vi "_FPGA Wait.vi"(4 "error in":errorcluster, 5 "Timeout (2000ms)":u32=2000, 6 "Indicator":T1=enum."Ready") -> (0 "error out":errorcluster)   [LabVIEW 2012]
uses:
  Type/_FPGA Indicator.ctl
  Type/_RW Status.ctl
  Type/_LED States.ctl
  _RT Global.vi
  <vilib>/Utility/error.llb/Error Cluster From Error Code.vi
  <vilib>/rvi/errors/niLvFpgaAdjustHostInterfaceError.vi
  <vilib>/rvi/interface/nirviReadWriteControl/nirviReadWriteControl.xnode
  FPGA Bitfiles/FPGA9606.lvbitx
  NiFpgaLv.dll
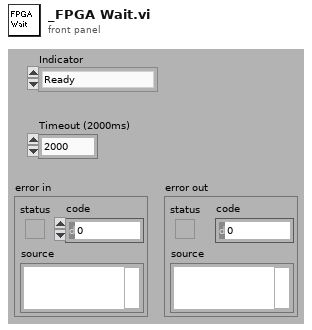
[diagram p1: front panel]
types:
  T1 = typedef "_FPGA Indicator.ctl" = enum16{"Done", "Ready", "Count Available", "SendSerial", "LED State"}
  T2 = typedef "_RW Status.ctl" = enum8{"Done", "Do Read", "Do Write", "Set Latch1", "Set Latch2", "Set Latch3", "Set Latch4", "RP ON", "EL ON", "Serial Send", "Set LC Out", "Get LC In", "Read VAC", "Table Test", "Get Interlock", "Do Read2", "Do Write2"}
  T3 = typedef "_LED States.ctl" = enum8{"Idle", "Solid B", "Solid R", "Solid P", "Off B", "Off R", "Off P", "Off BRP", "Off RP", "Flash R&P", "Flash P"}
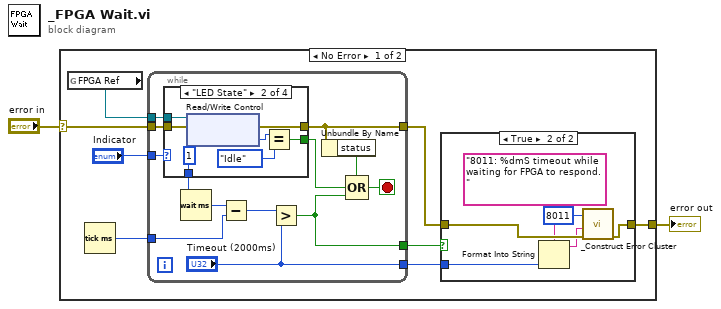
[diagram p0: block diagram]
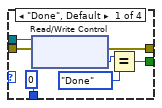
[diagram p3: hidden frame]
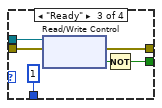
[diagram p4: hidden frame]
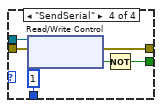
[diagram p5: hidden frame]
diagram:
  n1 = case shown="No Error" "error in" {
    selector: "error in" -> [w5 w56]
    tunnel: [w7 w56] -> w2
    frame No Error {
      n2 = global read "_RT Global.vi" "FPGA Ref"() -> (w3:refnum<k20>)
      n3 = Tick Count (ms)() -> (millisecond timer value=w10:u32)
      n4 = while {
        tunnel: w3 -> [w29]
        tunnel: w5 -> [w28]
        tunnel: [w20] -> w8
        tunnel: w10 -> [w27]
        tunnel: [w23] -> w9
        tunnel: "Indicator" -> [w22]
        tunnel: ["Timeout (2000ms)"] -> w4
        stop <- w24 stop-if-true
        n5 = case shown="\"LED State\"" w22 {
          tunnel: w29 -> [w36 w43 w49 w55]
          tunnel: w28 -> [w35 w42 w48 w54]
          tunnel: [w34 w41 w47 w53] -> w20
          tunnel: [w33 w40 w45 w51] -> w25
          tunnel: [u32 0 ("milliseconds to wait") u32 1 ("milliseconds to wait") u32 1 ("milliseconds to wait") u32 1 ("milliseconds to wait")] -> w17
          frame "Done", Default {
            n6 = xnode "Read/Write Control"("FPGA VI Reference In"=w36, "error in"=w35) -> ("error out"=w34:errorcluster, "R/W Status"=w32:T2)  [unwired: 1 out]
            n7 = Equal?(x=w32, y=_RW_Status."Done" ("R/W Status")) -> (x = y?=w33:bool)
          }
          frame "LED State" {
            n8 = xnode "Read/Write Control"("FPGA VI Reference In"=w43, "error in"=w42) -> ("error out"=w41:errorcluster, "LED States"=w39:T3)  [unwired: 1 out]
            n9 = Equal?(x=w39, y=_LED_States."Idle" ("R/W Status")) -> (x = y?=w40:bool)
          }
          frame "Ready" {
            n10 = xnode "Read/Write Control"("FPGA VI Reference In"=w49, "error in"=w48) -> ("error out"=w47:errorcluster, "Running"=w46:bool)  [unwired: 1 out]
            n11 = Not(x=w46) -> (.not. x?=w45:bool)
          }
          frame "SendSerial" {
            n12 = xnode "Read/Write Control"("FPGA VI Reference In"=w55, "error in"=w54) -> ("error out"=w53:errorcluster, "Send Serial"=w52:bool)  [unwired: 1 out]
            n13 = Not(x=w52) -> (.not. x?=w51:bool)
          }
        }
        n14 = Wait (ms)(milliseconds to wait=w17) -> (millisecond timer value=w18:u32)
        n15 = Subtract(x=w18, y=w27) -> (x-y=w26:u32)
        n16 = Greater?(x=w26, y="Timeout (2000ms)") -> (0:w23:bool)
        n17 = Unbundle By Name(w20) -> ("status"=w19:bool)
        n18 = Compound Arithmetic op=OR(w19, w25, w23) -> (w24:bool)
      }
      n19 = case shown="True" w9 {
        tunnel: w8 -> [_ w16]
        tunnel: [_ w15] -> w7
        tunnel: w4 -> [_ w12]
        frame False {
        }
        frame True {
          n20 = Format Into String(format string="8011: %dmS timeout while waiting for FPGA to respond.", w12) -> (resulting string=w13:string)  [unwired: 2 in, 1 out]
          n21 = call "_Construct Error Cluster.vi"("error in"=w16, "reason"=w13, "errorCode"=8011) -> ("error out"=w15:errorcluster)  [unwired: 1 in, 3 out]
        }
      }
    }
    frame Error {
    }
  }
  "error out" <- w2
